vi "tlacitkoOK.vi"(11 "NXT/EV3":T1) -> (0 "Boolean":bool, 3 "NXT/EV3 2":T1)   [LabVIEW 2013]
uses:
  <vilib>/NXT/Subs/LVHSConnector.ctl
  <vilib>/NXT/LegoClasses/BrickReference/BrickReference.lvclass
  <vilib>/NXT/Block Support/NXT_ButtonSelector.ctl
  <vilib>/NXT/Dual Mode Library/Sensors/readNXTButton.vi
  <vilib>/NXT/Dual Mode Library/Advanced/NXTFlag_Get_Integer.vi
  <vilib>/NXT/Dual Mode Library/Sensors/EV3_Infrared_Remote.vi
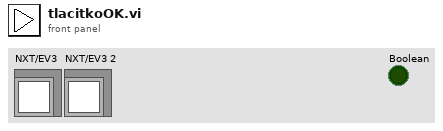
[diagram p1: front panel]
types:
  T1 = typedef "LVHSConnector.ctl" = refnum<class "BrickReference.lvclass">
  T2 = typedef "NXT_ButtonSelector.ctl" = u16
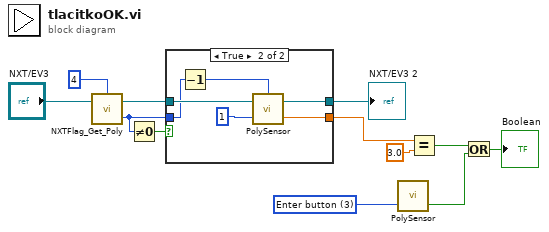
[diagram p0: block diagram]
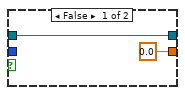
[diagram p2: hidden frame]
diagram:
  w10 = T2 3 items=["Enter button"=3, "Left button"=2, "Right button"=1, "Up Button"=4, "Down Button"=5] ("Button (Enter button)")
  n1 = call-poly <vilib>:"NXTFlag_Get_Poly.vi"("NXT/EV3"="NXT/EV3", "NXT/EV3 Flag Number"=4) -> ("Flag Value"=w1:i32, "NXT/EV3"=w6:T1)  [unwired: 1 in]
  n2 = Not Equal To 0?(x=w1) -> (x != 0?=w5:bool)
  n3 = case shown="True" w5 {
    tunnel: [sgl 0.0 ("Button Detected") w20] -> w12
    tunnel: w6 -> [w13 w18]
    tunnel: [w13 w17] -> w3
    tunnel: w1 -> [_ w15]
    frame False {
    }
    frame True {
      n4 = Decrement(x=w15) -> (x-1=w16:i32)
      n5 = call-poly <vilib>:"PolySensor.vi"("Channel"=u8 1, "NXT/EV3"=w18, "Port (Port 1)"=w16) -> ("Button Detected"=w20:sgl, "NXT/EV3"=w17:T1)
    }
  }
  "NXT/EV3 2" <- w3
  n6 = call-poly <vilib>:"PolySensor.vi"("Button (Enter button)"=w10) -> ("Yes/No"=w7:bool)  [unwired: 2 in, 1 out]
  n7 = Equal?(x=w12, y=sgl 3.0) -> (x = y?=w8:bool)
  n8 = Or(x=w8, y=w7) -> (x .or. y?=→"Boolean":bool)
